vi "08-send-and-receive-img.vi"() -> ()   [LabVIEW 2018, in "LV-0mq-Julia_roundtrip-lib.lvlib" / "LV2Julia_examples.lvlib"]
uses:
  LV2Julia_examples.lvlib
  LV2Julia_core/VIs/Server or client state.ctl
  LV2Julia_core/VIs/Commands.ctl
  f9264f0d-2c2d-4a22-a0da-9e005a3dfb77.vi
  f9264f0d-2c2d-4a22-a0da-9e005a3dfb77.vi/f9b6f95b-0c0d-4639-901d-5010536ce663.vi
  f9264f0d-2c2d-4a22-a0da-9e005a3dfb77.vi/f9b6f95b-0c0d-4639-901d-5010536ce663.vi/4382a19f-18e0-420b-a409-7d40f14172ac.vi
  f9264f0d-2c2d-4a22-a0da-9e005a3dfb77.vi/f9b6f95b-0c0d-4639-901d-5010536ce663.vi/318e2cdc-578f-46f6-91c8-6c060315616b.vi
  f9264f0d-2c2d-4a22-a0da-9e005a3dfb77.vi/f9b6f95b-0c0d-4639-901d-5010536ce663.vi/daa9cabe-c25e-4572-9c14-214e554045b4.vi
  LV2Julia_core/VIs/jl-scripts path.vi
  <vilib>/Utility/error.llb/Error Cluster From Error Code.vi
  LV2Julia_core/VIs/check ID validity.vi
  LV2Julia_core/VIs/bindata_descr to JSON.vi
  LV2Julia_core/VIs/check cluster field names.vi
  LV2Julia_core/VIs/concat JSON.vi
  LV2Julia_core/VIs/build request.vi
  LV2Julia_core/VIs/Parse server response.vi
  LV2Julia_core/VIs/log jl exceptions.vi
  <vilib>/ErrorRing/Error Ring.xnode
  LV2Julia_core/LV2Julia_core.lvlib
panel:
  in  "Transform":T1
  out "picture sent":picture
  in  "image file path":path=path "../other_files/peppers_color_256.png"
  out "picture received":picture
  out "short error info":string
  in  "next":bool
  out "current error":errorcluster
  out "final error":errorcluster
  in  "stop":bool
  out "ZMQ timeout":bool
  out "Julia script file path":path
  out "temporary script path":path
  out "Jl Server state":T2
  # "If you don't see any received picture. check the scrollbars!"
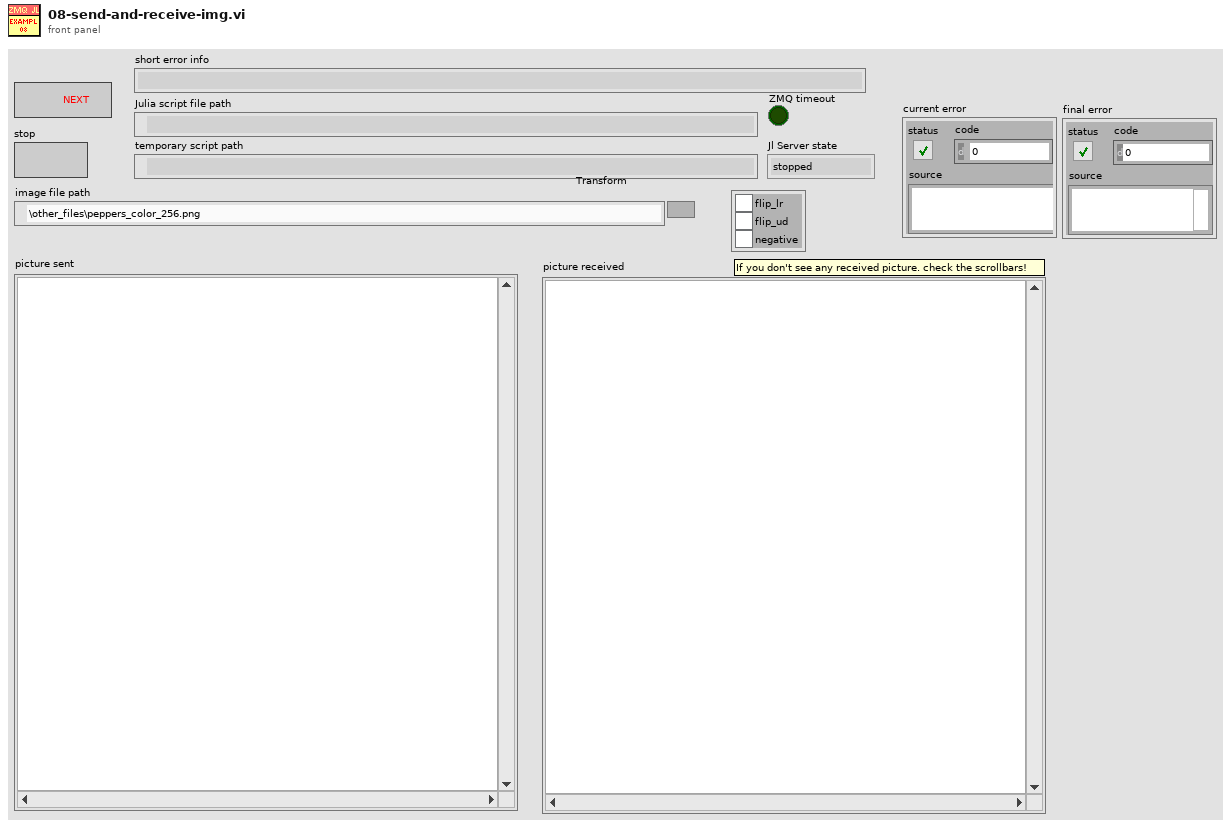
[diagram p1: front panel]
types:
  T1 = cluster{"flip_lr":bool, "flip_ud":bool, "negative":bool}
  T2 = typedef "LV-0mq-Julia_roundtrip-lib.lvlib/LV2Julia_core.lvlib/Server or client state.ctl" = enum16{"stopped", "running", "unknown"}
  T3 = typedef "LV-0mq-Julia_roundtrip-lib.lvlib/LV2Julia_core.lvlib/Commands.ctl" = enum16{"Start Jl-server & Init LV-client", "Send request & Get response ", "Stop Jl-server & Cleanup LV-client", "Cleanup LV-client", "Start Jl-server", "Stop Jl-server", "Init LV-Client", "Cleanup LV-Client", "(not allowed)", "Set LV Client state", "Set Jl Server state", "set ZMQ timeout", "read ZMQ timeout", "read-out state"}
  T4 = typedef "imagedata.ctl" = cluster{"image type":i32, "image depth":i32, "image":u8[], "mask":u8[], "colors":u32[], "Rectangle":cluster{"left":i16, "top":i16, "right":i16, "bottom":i16}}
  T5 = typedef "LV-0mq-Julia_roundtrip-lib.lvlib/LV2Julia_core.lvlib/Bindata&description.ctl" = cluster{"bindata_descr":T6[], "bindata":u8[]}
  T6 = typedef "LV-0mq-Julia_roundtrip-lib.lvlib/LV2Julia_core.lvlib/Bindata description.ctl" = cluster{"nofbytes":i32, "numtype":string, "start":i32, "arrdims":i32[], "kwarg_name":string, "category":string}
  T7 = typedef "LV-0mq-Julia_roundtrip-lib.lvlib/LV2Julia_core.lvlib/detailed error info.ctl" = cluster{"exception_or_info":string, "trace":T8[]}
  T8 = typedef "LV-0mq-Julia_roundtrip-lib.lvlib/LV2Julia_core.lvlib/StackFrame.ctl" = cluster{"frame_summary":string, "func":string, "linfo":string, "file":string, "line":i32, "pointer":u64, "from_c":bool, "inlined":bool}
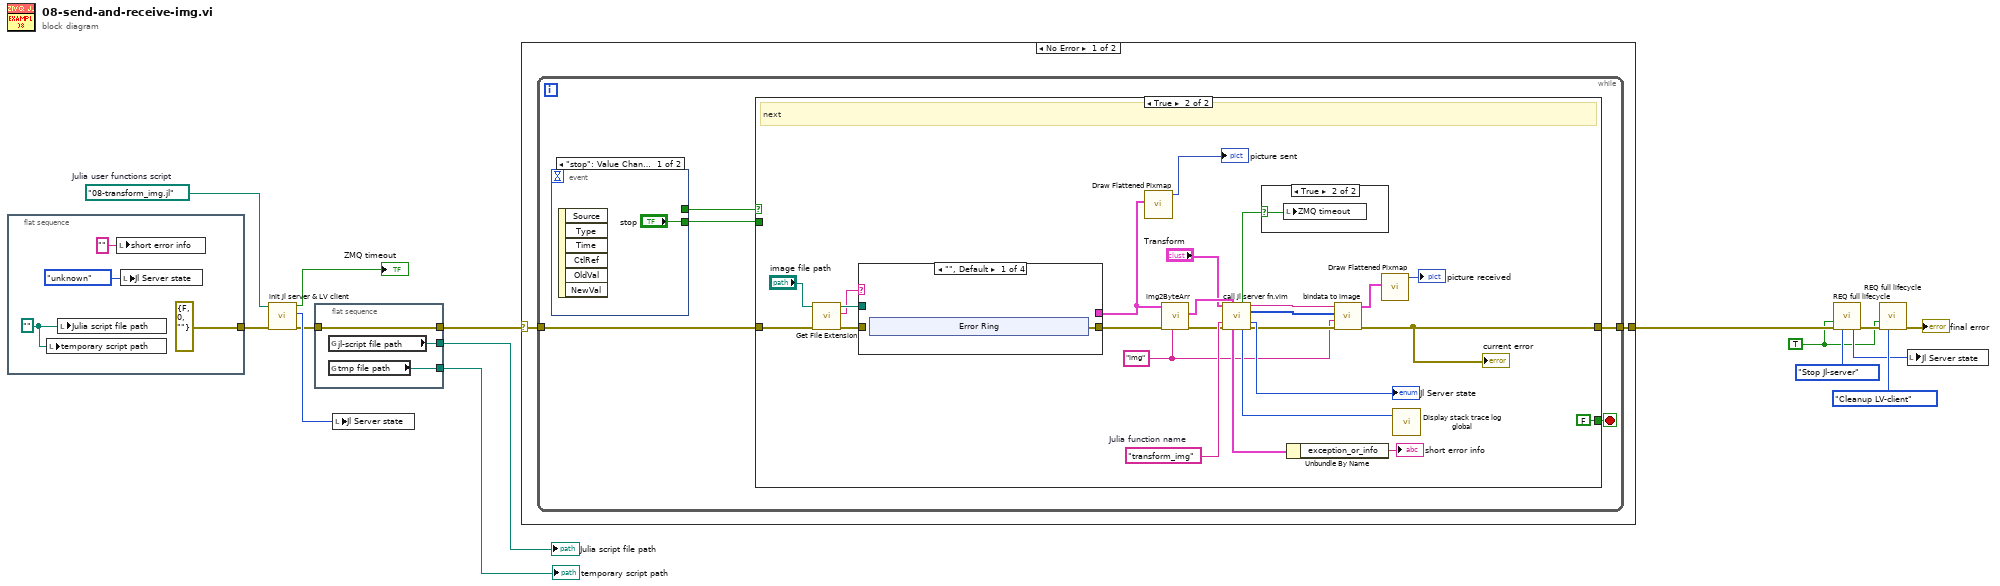
[diagram p0: block diagram]
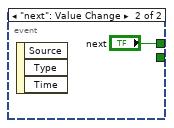
[diagram p2: hidden frame]
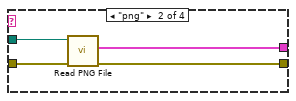
[diagram p4: hidden frame]
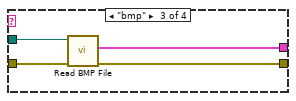
[diagram p5: hidden frame]
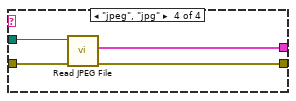
[diagram p6: hidden frame]
diagram:
  w3 = path "08-transform_img.jl"  # Julia user functions script
  w6 = TRUE ("Force command")
  n1 = flat-sequence {
    tunnel: [errorcluster {"status"=FALSE, "code"=0, "source"=""} ("error in (no error)")] -> w2
    frame #0 {
      w17 = path ""
      n2 = local write "temporary script path"(w17) -> ()
      n3 = local write "Julia script file path"(w17) -> ()
      n4 = local write "short error info"("" ("short error info")) -> ()
      n5 = local write "Jl Server state"(Server_or_client_state."unknown" ("Jl Server state out")) -> ()
    }
  }
  n6 = call "init Jl server & LV client.vi"("error in (no error)"=w2, "Julia user functions script"=w3) -> ("error out"=w1:errorcluster, "Jl Server state out"=w4:T2, "timeout?"=→"ZMQ timeout":bool)  [unwired: 7 in]
  n7 = flat-sequence {
    tunnel: [w22] -> w10
    tunnel: w1 -> [w22]
    tunnel: [w21] -> w8
    tunnel: [w20] -> w9
    frame #0 {
      n8 = global read "jl-scripts path.vi" "jl-script file path"() -> (w21:path)
      n9 = global read "jl-scripts path.vi" "tmp file path"() -> (w20:path)
    }
  }
  n10 = local write "Jl Server state"(w4) -> ()
  n11 = case shown="No Error" w10 {
    selector: w10 -> [w23 w78]
    tunnel: [w24 w78] -> w15
    frame No Error {
      n12 = while {
        tunnel: w23 -> [w28]
        tunnel: [w29] -> w24
        stop <- w26 stop-if-true
        n13 = event shown="[0] \"stop\": Value Change" {
          selector: _ -> [_ _]
          dyn-events: _ -> [_ _]
          timeout: _ -> [_ _]
          tunnel: [_ "next"] -> w27
          tunnel: ["stop" _] -> w25
          event "stop": Value Change {
            n14 = event-data() -> ()  [unwired: 1 in, 6 out]
          }
          event "next": Value Change {
            n15 = event-data() -> ()  [unwired: 1 in, 3 out]
          }
        }
        n16 = case shown="True" w27 {
          tunnel: [w33 w48] -> w29
          tunnel: w28 -> [w33 w39]
          tunnel: [w32 FALSE ("stop this VI only")] -> w26
          tunnel: w25 -> [w32 _]
          frame False {
            # "stop"
          }
          frame True {
            w37 = "img" ("name")
            w57 = "transform_img"  # Julia function name
            # "next"
            n17 = call <vilib>:"Get File Extension.vi"("error in (no error)"=w39, "file"="image file path") -> ("error out"=w42:errorcluster, "lowercase file extension"=w40:string, "dup file"=w43:path)  [unwired: 5 in, 2 out]
            n18 = case shown="\"\", Default" w40 {
              tunnel: [_ w68 w72 w76] -> w45
              tunnel: w43 -> [_ w67 w71 w75]
              tunnel: w42 -> [_ w66 w70 w74]
              tunnel: [w59 w65 w69 w73] -> w41
              frame "", Default {
                n19 = xnode "Error Ring"() -> ("error out"=w59:errorcluster)
              }
              frame "png" {
                n20 = call <vilib>:"Read PNG File.vi"("error in (no error)"=w66, "path to PNG file"=w67) -> ("error out"=w65:errorcluster, "image data"=w68:T4)  [unwired: 7 in, 1 out]
              }
              frame "bmp" {
                n21 = call <vilib>:"Read BMP File.vi"("error in (no error)"=w70, "path to BMP file"=w71) -> ("error out"=w69:errorcluster, "image data"=w72:T4)  [unwired: 7 in, 1 out]
              }
              frame "jpeg", "jpg" {
                n22 = call <vilib>:"Read JPEG File.vi"("error in (no error)"=w74, "path to JPEG file"=w75) -> ("error out"=w73:errorcluster, "image data"=w76:T4)  [unwired: 7 in, 1 out]
              }
            }
            n23 = call <vilib>:"Draw Flattened Pixmap.vi"("image data"=w45) -> ("new picture"=→"picture sent":picture)  [unwired: 8 in]
            n24 = call "img2ByteArr.vi"("kwarg_name"=w37, "error in (no error)"=w41, "img in"=w45) -> ("error out"=w38:errorcluster, "Bindata & descr out"=w35:T5)  [unwired: 6 in, 1 out]
            n25 = call "call Jl server fn.vim"("Arguments 1"="Transform", "Bindata & descr in"=w35, "fun2call"=w57, "error in (no error)"=w38) -> ("timeout?"=w55:bool, "JSON received"=w47:string, "binary data received"=w46:u8[], "Jl Server state out"=→"Jl Server state":T2, "detailed error info"=w53:T7, "return code"=w54:u8, "error out"=w49:errorcluster)  [unwired: 5 in]
            n26 = case shown="True" w55 {
              selector: w55 -> [_ w77]
              frame False {
              }
              frame True {
                n27 = local write "ZMQ timeout"(w77) -> ()
              }
            }
            n28 = Unbundle By Name(w53) -> ("exception_or_info"=→"short error info":string)
            n29 = call "bindata to image.vi"("error in (no error)"=w49, "name"=w37, "binary data in"=w46, "JSON in"=w47) -> ("error out"=w48:errorcluster, "img out"=w50:T4)  [unwired: 6 in]
            "current error" <- w48
            n30 = call <vilib>:"Draw Flattened Pixmap.vi"("image data"=w50) -> ("new picture"=→"picture received":picture)  [unwired: 8 in]
            n31 = call "Display stack trace log global.vi"("server return code"=w54) -> ()  [unwired: 3 in]
          }
        }
      }
    }
    frame Error {
    }
  }
  n32 = call "REQ full lifecycle.vi"("Force command"=w6, "error in"=w15, "command"=Commands."Stop Jl-server") -> ("Jl Server state out"=w7:T2, "error out"=w13:errorcluster)  [unwired: 6 in, 5 out]
  n33 = call "REQ full lifecycle.vi"("Force command"=w6, "error in"=w13, "command"=Commands."Cleanup LV-client") -> ("error out"=→"final error":errorcluster)  [unwired: 6 in, 6 out]
  n34 = local write "Jl Server state"(w7) -> ()
  "temporary script path" <- w9
  "Julia script file path" <- w8
